vi "FTW-Container-QueryValue.vi"(0 "Container":refnum<class "FTW-Container.lvclass">, 5 "Type and Defaults":variant, 11 "error in":errorcluster) -> (4 "Container out":refnum<class "FTW-Container.lvclass">, 6 "Result":variant, 15 "error out":errorcluster)   [LabVIEW 2014, in "FTW-Container.lvclass"]
uses:
  FTW-Container.lvclass
panel:
  # "Inputs"
  # "Outputs"
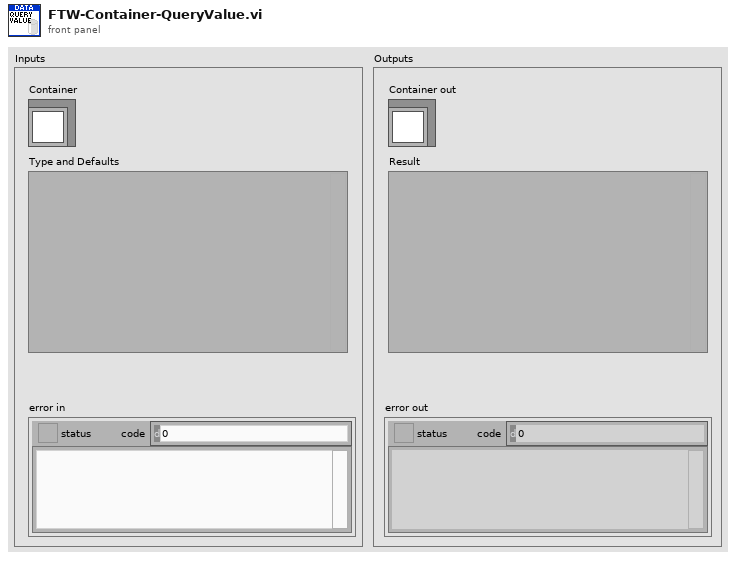
[diagram p1: front panel]
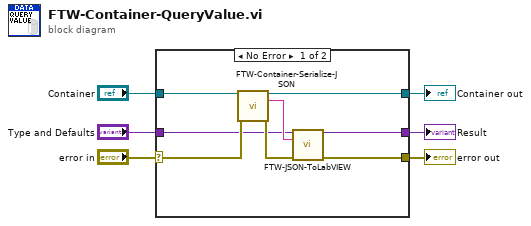
[diagram p0: block diagram]
diagram:
  n1 = case shown="No Error" "error in" {
    selector: "error in" -> [w11 w17]
    tunnel: [w7 w17] -> w6
    tunnel: "Container" -> [w14 w16]
    tunnel: [w13 w16] -> w3
    tunnel: "Type and Defaults" -> [w9 w15]
    tunnel: [w8 w15] -> w1
    frame No Error {
      n2 = call "FTW-Container-Serialize-JSON.vi"("Container"=w14, "error in"=w11) -> ("Container out"=w13:refnum<class "FTW-Container.lvclass">, "Serialized Container"=w12:string, "error out"=w10:errorcluster)  [unwired: 11 in]
      n3 = call "FTW-JSON-ToLabVIEW.vi"("Type and Defaults"=w9, "JSON String"=w12, "error in"=w10) -> ("Populated Values"=w8:variant, "error out"=w7:errorcluster)  [unwired: 11 in]
    }
    frame Error {
    }
  }
  "error out" <- w6
  "Container out" <- w3
  "Result" <- w1
